vi "create file for writing to.vi"(7 "Queues":T1, 11 "fileIO":T2) -> (2 "Byte Stream File out":refnum<file>, 3 "fileIO out":T2, 5 "target filename":path)   [LabVIEW 2018]
uses:
  type defs/file IO data.ctl
  type defs/channelControl.ctl
  RT/Type Defs/channelScalingTypes.ctl
  RT/Type Defs/scalingMethods.ctl
  ICL-LabVIEW_General/data channels/parent class/Data Channel.lvclass
  type defs/Queues.ctl
  supporting VIs/polymorphic VIs/enqueue for user interface.vi
  ICL-LabVIEW_General/data channels/data channels.lvlib
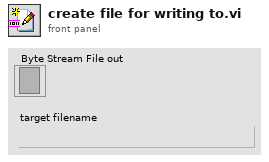
[diagram p1: front panel]
types:
  T1 = typedef "Queues.ctl" = cluster{"messageHandler":refnum<queue>, "comms":refnum<queue>, "dataStream":refnum<queue>, "dataProcessor":refnum<queue>, "fileIO":refnum<queue>, "userInterface":refnum<queue>, "errors":refnum<queue>, "customCompressor":refnum<queue>}
  T2 = typedef "file IO data.ctl" = cluster{"params":cluster{"startFolder":path, "channelConfigPath":path}, "vars":cluster{"channelConfig ":T3[], "writing":cluster{"streaming":bool, "fixedLength":bool, "pointCount":u32, "timeZero":dbl, "pointsWritten":u32, "dataRate":u16}, "channelCount":u16, "fileTarget":cluster{"Save folder":path, "Target filename":string, "file ref":refnum<file>, "pulsatorSpeed":string, "motorSpeed":string, "valvePosition":string, "torqueFilter":bool, "pulsatorRunning":bool, "motorRunning":bool}, "channels":refnum<class "Data Channel.lvclass">[]}}
  T3 = typedef "channelControl.ctl" = cluster{"index":u16, "active":bool, "channelType":T4, "module":u16, "terminal":u16, "channelName":string, "scalingMethod":T5, "scalingParameters":dbl[], "scaledUnits":string, "tempOffset":dbl}
  T4 = typedef "channelScalingTypes.ctl" = enum16{"calculation", "measurement", "scanivalve", "output", "digital"}
  T5 = typedef "scalingMethods.ctl" = enum16{"none", "linear", "thermocouple", "polynomial", "encoder", "RTD"}
  T6 = enum16{"open", "replace", "create", "open or create", "replace or create", "replace or create with confirmation"}
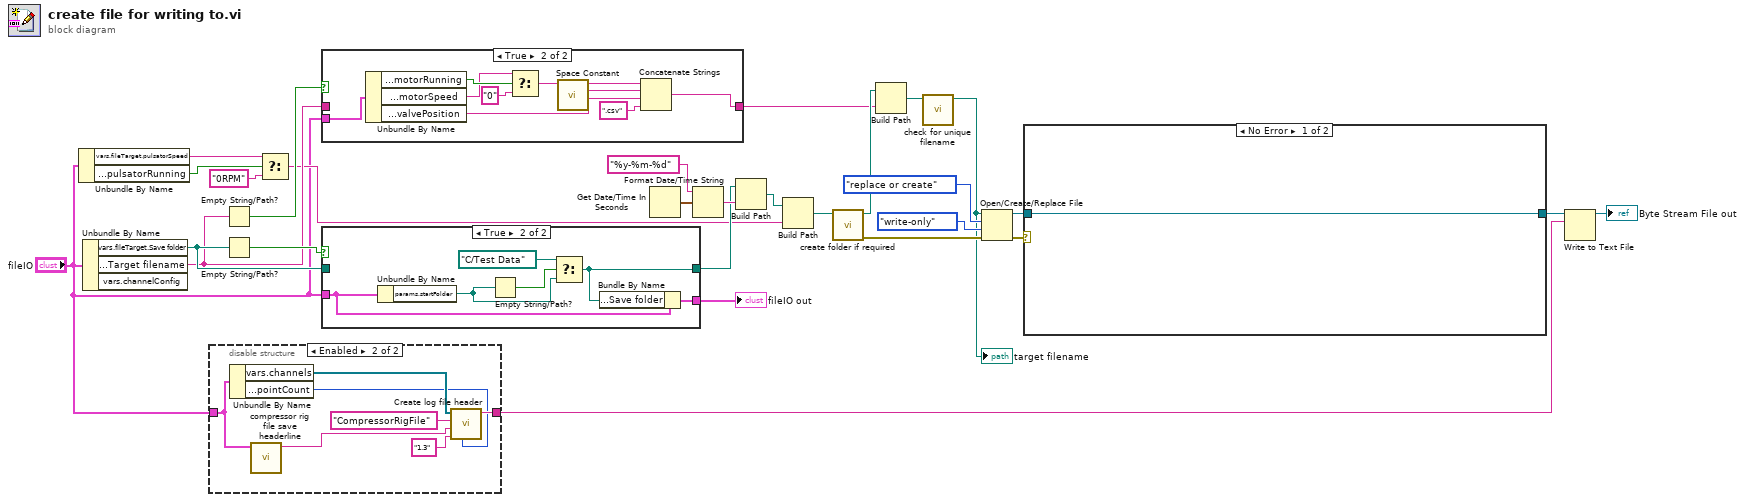
[diagram p0: block diagram]
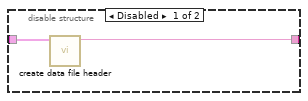
[diagram p2: hidden frame]
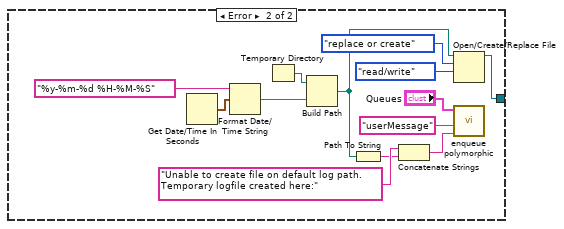
[diagram p3: hidden frame]
diagram:
  n1 = Unbundle By Name("fileIO") -> ("vars.fileTarget.pulsatorSpeed"=w3:string, "vars.fileTarget.pulsatorRunning"=w5:bool)
  n2 = Unbundle By Name("fileIO") -> ("vars.fileTarget.Save folder"=w25:path, "vars.fileTarget.Target filename"=w23:string)  [unwired: 1 out]
  n3 = disable-structure shown="Enabled" {
    disable-tunnel: [w30 w37] -> w20
    disable-tunnel: "fileIO" -> [w29 w31]
    frame Disabled {
      n4 = call "create data file header.vi"("fileIO"=w29) -> ("header string"=w30:string)  [unwired: 10 in]
    }
    frame Enabled {
      n5 = Unbundle By Name(w31) -> ("vars.channels"=w33:refnum<class "Data Channel.lvclass">[], "vars.writing.pointCount"=w32:u32)
      n6 = call "compressor rig file save headerline.vi"("fileIO"=w31) -> ("compressorRig save file headerline"=w36:string)  [unwired: 10 in]
      n7 = call "Create log file header.vi"("dataPoints"=w32, "custom logfile version"="1.3", "custom logfile header line"=w36, "custom file title"="CompressorRigFile", "dataChannels"=w33) -> ("header string"=w37:string)  [unwired: 6 in]
    }
  }
  n8 = Empty String/Path?(string/path=w23) -> (empty?=w24:bool)
  n9 = Empty String/Path?(string/path=w25) -> (empty?=w26:bool)
  n10 = Select(t=w3, s=w5, f="0RPM") -> (s? t:f=w2:string)
  n11 = case shown="True" w24 {
    tunnel: w23 -> [w38 _]
    tunnel: [w38 w44] -> w7
    tunnel: "fileIO" -> [_ w47]
    frame False {
    }
    frame True {
      n12 = Unbundle By Name(w47) -> ("vars.fileTarget.motorRunning"=w42:bool, "vars.fileTarget.motorSpeed"=w41:string, "vars.fileTarget.valvePosition"=w46:string)
      n13 = Select(t=w41, s=w42, f="0") -> (s? t:f=w40:string)
      n14 = call <vilib>:"Space Constant.vi"() -> ("String"=w45:string)
      n15 = Concatenate Strings(w40, w45, w46, ".csv" ("string")) -> (w44:string)
    }
  }
  n16 = case shown="True" w26 {
    tunnel: "fileIO" -> [w49 w55]
    tunnel: [w49 w54] -> w22
    tunnel: w25 -> [w48 _]
    tunnel: [w48 w50] -> w12
    frame False {
    }
    frame True {
      n17 = Unbundle By Name(w55) -> ("params.startFolder"=w52:path)
      n18 = Empty String/Path?(string/path=w52) -> (empty?=w53:bool)
      n19 = Select(t=path "C:/Test Data", s=w53, f=w52) -> (s? t:f=w50:path)
      n20 = Bundle By Name(cluster=w55, "vars.fileTarget.Save folder"=w50) -> (w54:T2)
    }
  }
  "fileIO out" <- w22
  n21 = Get Date/Time In Seconds() -> (seconds since 1Jan1904=w15:timestamp)
  n22 = Format Date/Time String(time format string (%c)="%y-%m-%d", seconds (now)=w15) -> (date/time string=w13:string)  [unwired: 1 in]
  n23 = Build Path(base path=w12, name or relative path=w13) -> (appended path=w9:path)
  n24 = Build Path(base path=w9, name or relative path=w2) -> (appended path=w8:path)
  n25 = call "create folder if required.vi"("folder path"=w8) -> ("error out"=w11:errorcluster, "actual path"=w10:path)  [unwired: 9 in]
  n26 = Build Path(base path=w10, name or relative path=w7) -> (appended path=w21:path)
  n27 = call "check for unique filename.vi"("filename"=w21) -> ("unique filename"=w6:path)  [unwired: 10 in]
  "target filename" <- w6
  n28 = Open/Create/Replace File(file path (use dialog)=w6, error in=w11, operation (0:open)=T6."replace or create", access (0:read/write)=enum16{"read/write", "read-only", "write-only"}."write-only") -> (refnum out=w17:refnum<file>, error out=w18:errorcluster)  [unwired: 2 in, 1 out]
  n29 = case shown="No Error" w18 {
    tunnel: w17 -> [w56 _]
    tunnel: [w56 w68] -> w16
    frame No Error {
    }
    frame Error {
      n30 = Get Date/Time In Seconds() -> (seconds since 1Jan1904=w59:timestamp)
      n31 = Format Date/Time String(time format string (%c)="%y-%m-%d %H-%M-%S", seconds (now)=w59) -> (date/time string=w57:string)  [unwired: 1 in]
      n32 = Temporary Directory() -> (w69:path)
      n33 = Build Path(base path=w69, name or relative path=w57) -> (appended path=w62:path)
      n34 = Path To String(path=w62) -> (string=w61:string)
      n35 = Concatenate Strings("Unable to create file on default log path. Temporary logfile created here:", w61) -> (w60:string)
      n36 = Open/Create/Replace File(file path (use dialog)=w62, operation (0:open)=T6."replace or create", access (0:read/write)=enum16{"read/write", "read-only", "write-only"}."read/write") -> (refnum out=w68:refnum<file>)  [unwired: 3 in, 2 out]
      n37 = call-poly "enqueue polymorphic.vi"("data"=w60, "message"="userMessage", "Queues"="Queues") -> ()  [unwired: 8 in, 1 out]
    }
  }
  n38 = Write to Text File(file (use dialog)=w16, text=w20) -> (refnum out=→"Byte Stream File out":refnum<file>)  [unwired: 2 in, 2 out]
